vi "FilterEMGSignal.vi"(9 "Data":dynamicdata(waveform), 10 "Upper Cut-Off":dbl=300.0, 11 "Lower Cut-Off":dbl=20.0) -> (3 "Waveform":waveform(dbl))   [LabVIEW 2016]
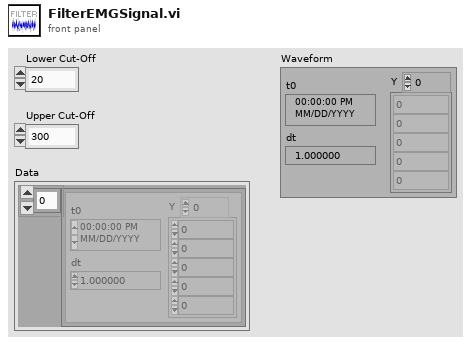
[diagram p1: front panel]
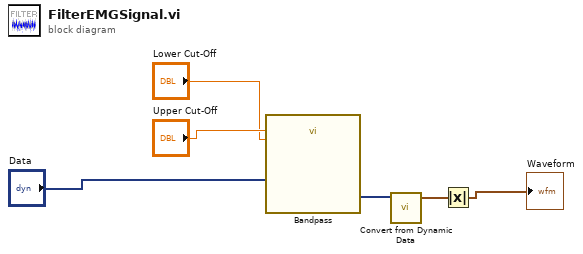
[diagram p0: block diagram]
diagram:
  n1 = call "Bandpass"("Lower Cut-Off"="Lower Cut-Off", "Upper Cut-Off"="Upper Cut-Off", "Signal"="Data") -> ("Filtered Signal"=w5:dynamicdata)  [unwired: 7 in, 1 out]
  n2 = call "Convert from Dynamic Data"("Dynamic Data Type"=w5) -> ("Waveform"=w4:waveform(dbl))  [unwired: 3 in]
  n3 = Absolute Value(x=w4) -> (abs(x)=→"Waveform":waveform(dbl))
